vi "yaw.vi"() -> ()   [LabVIEW 2009]
uses:
  <vilib>/rvi/FXPMathLib/FxpAtan2/XNode/nifxpmath_Atan2.xnode
  <vilib>/rvi/FXPMathLib/FxpAtan2/subVIs/nifxpmath_Atan2_SimConfig.ctl
  <vilib>/rvi/FXPMathLib/FxpAtan2/simVIs/DllFxpAtan2Temp_sub.vi
panel:
  out "yaw 2":dbl
  out "yaw":fxp<+/-,16,2> format="%.15g"
  in  "q3":i16
  in  "q2":i16
  in  "q1":i16
  in  "q0":i16
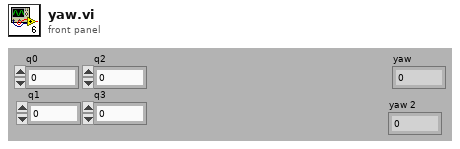
[diagram p1: front panel]
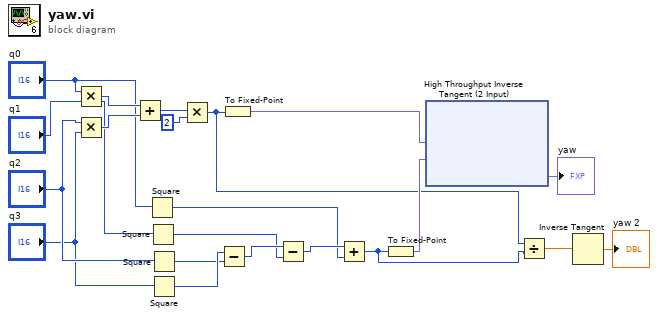
[diagram p0: block diagram]
diagram:
  n1 = Multiply(x="q0", y="q1") -> (x*y=w21:i16)
  n2 = Multiply(x="q2", y="q3") -> (x*y=w20:i16)
  n3 = Add(x=w21, y=w20) -> (x+y=w19:i16)
  n4 = Square(x="q0") -> (x^2=w8:i16)
  n5 = Square(x="q1") -> (x^2=w10:i16)
  n6 = Square(x="q2") -> (x^2=w11:i16)
  n7 = Square(x="q3") -> (x^2=w12:i16)
  n8 = Multiply(x=w19, y=i16 2) -> (x*y=w4:i16)
  n9 = Subtract(x=w12, y=w11) -> (x-y=w13:i16)
  n10 = To Fixed-Point(number=w4) -> (fixed-point=w6:fxp<+/-,16,16>)  [unwired: 1 in]
  n11 = Subtract(x=w13, y=w10) -> (x-y=w9:i16)
  n12 = Add(x=w9, y=w8) -> (x+y=w3:i16)
  n13 = To Fixed-Point(number=w3) -> (fixed-point=w5:fxp<+/-,16,16>)  [unwired: 1 in]
  n14 = xnode "High Throughput Inverse Tangent (2 Input)"("y"=w6, "x"=w5) -> ("atan2(y,x) (pi)"=→"yaw":fxp<+/-,16,2>)
  n15 = Divide(x=w4, y=w3) -> (x/y=w2:dbl)
  n16 = Inverse Tangent(1:w2) -> (0:→"yaw 2":dbl)
